vi "Omega DFG51-2 Force Gauge Logger.vi"() -> ()   [LabVIEW 2017]
uses:
  <vilib>/regexp/Match Regular Expression.xnode
  <vilib>/Analysis/NI_AALPro.lvlib
panel:
  out "after match":string
  out "before match":string
  in  "Tab Control":enum32{"Front Panel", "Save"}(tab)
  in  "Save?":bool=TRUE
  out "Realtime Plot":dbl(graph)
  out "Summary Plot":T1(graph)
  out "Device Response":string
  in  "Query to Device":string="?"
  in  "?":bool
  in  "Speed of Motor (cm/s)":dbl=0.01
  in  "COM Port":refnum<visa-resource-name>="COM5"
  out "Max Force":dbl format="%.4g"
  out "Integral of Force":dbl
  in  "Clear on Start":bool=TRUE
  out "Force vs. Displacement":cluster{"Get Start Time (s)":dbl, dbl, dbl[]}(graph)
  out "COM error out":errorcluster
  # "Molly's Palmer Stand = 0.01 cm/s = 6mm/min"
  # "Sample rate = 64 ms interval = 16Hz"
  # "8/31/2018\nMolly Roberts\n3/18/2015\nMatt George\nmngeorge@uw.edu"
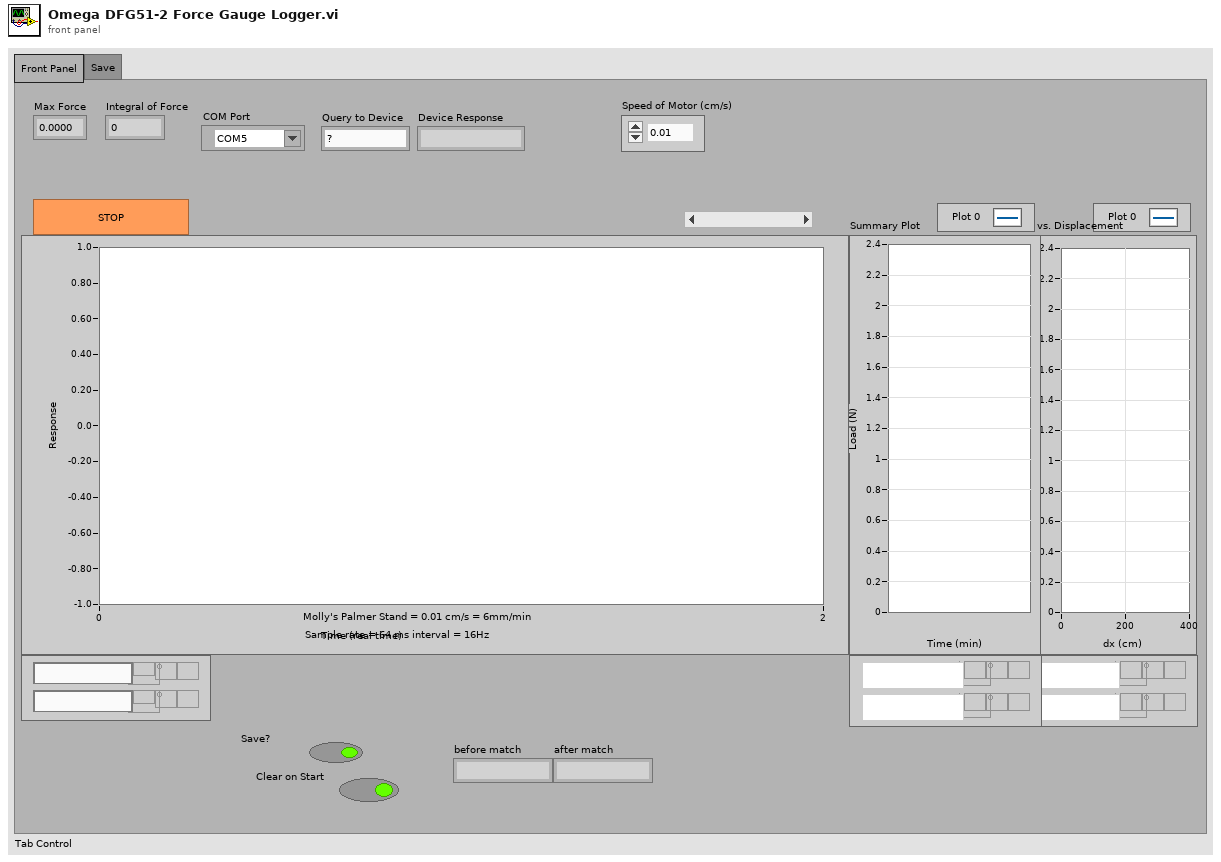
[diagram p1: front panel]
types:
  T1 = cluster{"Get Start Time (s)":dbl, "Sample rate (ms)":dbl, dbl[]}
  T2 = typedef "NI_Matrix.lvlib/RealMatrix.ctl" = dbl[][]
  T3 = enum16{"open", "replace", "create", "open or create", "replace or create", "replace or create with confirmation"}
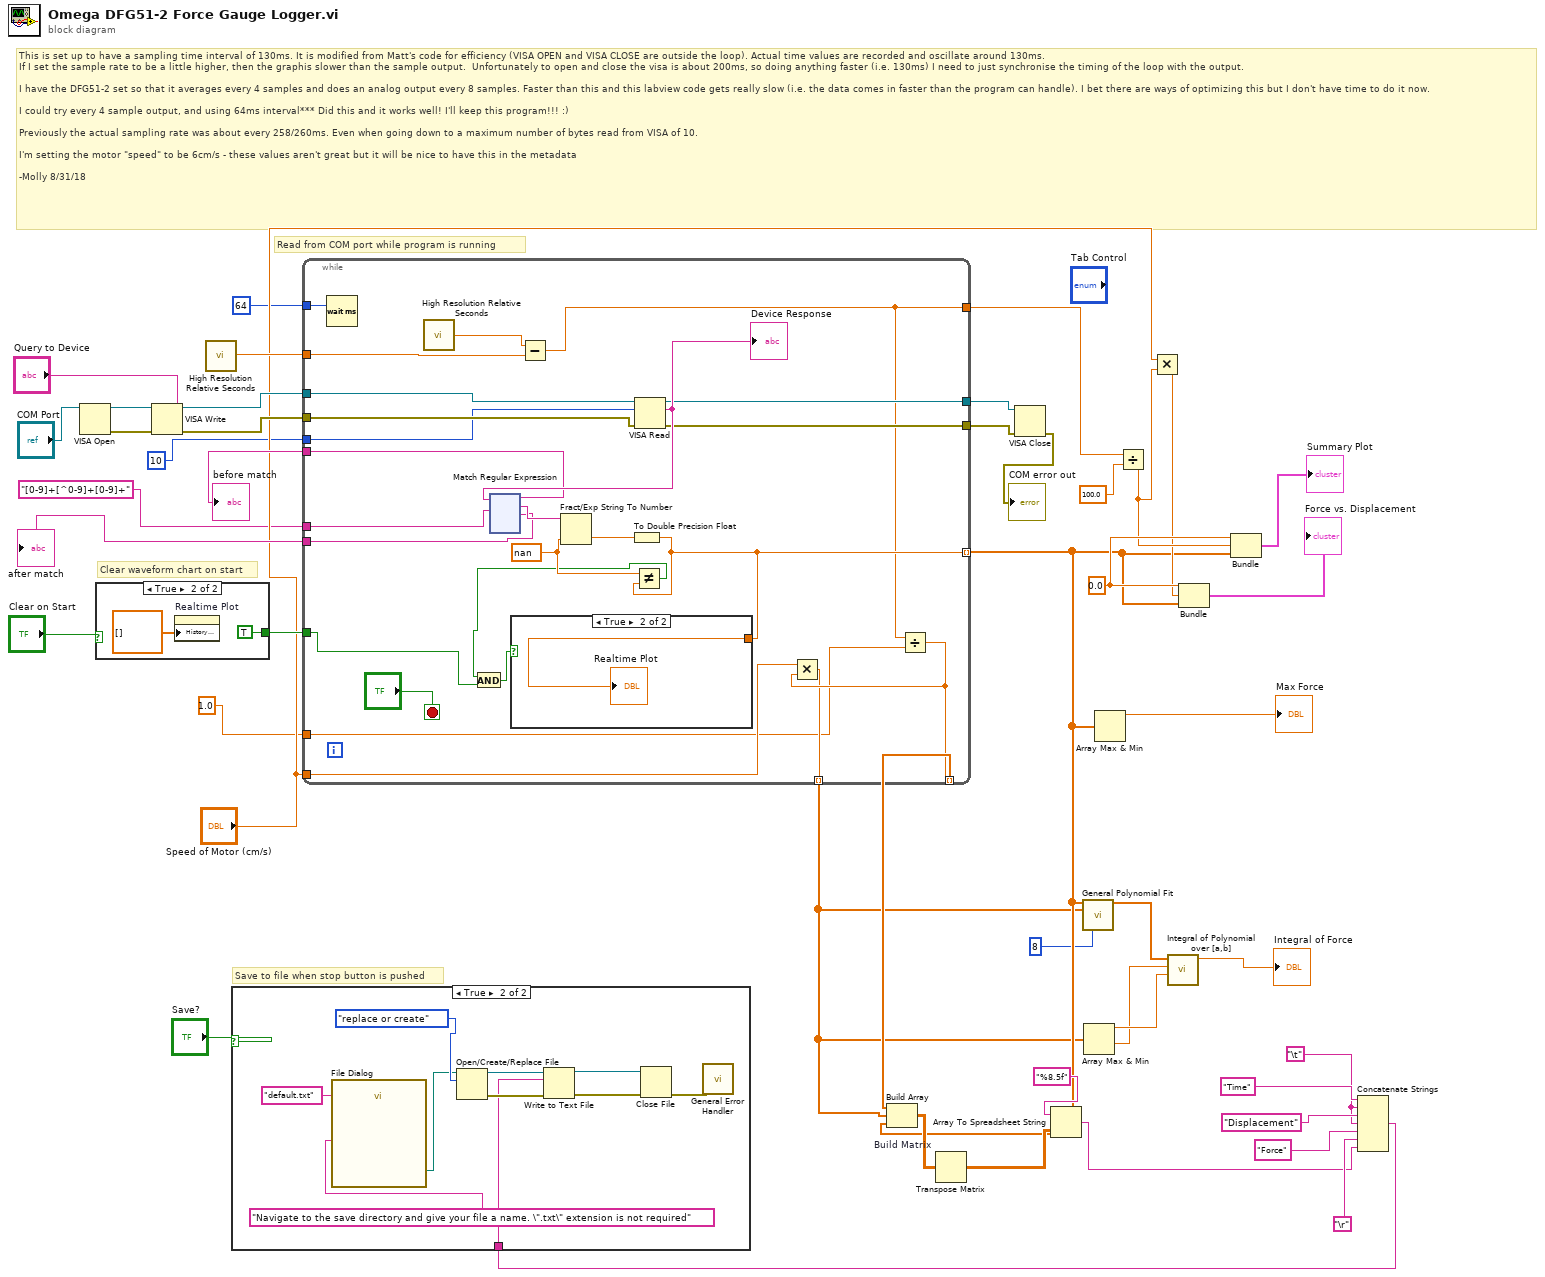
[diagram p0: block diagram]
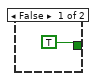
[diagram p2: hidden frame]
diagram:
  w35 = "\t"
  w45 = 0.0
  # "This is set up to have a sampling time interval of 130ms. It is modified from Matt's code for efficiency (VISA OPEN and VISA CLOSE are outside the loop). Actual time values are recorded and oscillate around 130ms. \nIf I set the sample rate to be a little higher, then the graphis slower than the sample output.  Unfortunately to open and close the visa is about 200ms, so doing anything faster (i.e. 130ms) I need to just synchronise the timing of the loop with the output. \n\nI have the DFG51-2 set so that it averages every 4 samples and does an analog output every 8 samples. Faster than this and this labview code gets really slow (i.e. the data comes in faster than the program can handle). I bet there are ways of optimizing this but I don't have time to do it now.\n\nI could try every 4 sample output, and using 64ms interval*** Did this and it works well! I'll keep this program!!! :)\n\nPreviously the actual sampling rate was about every 258/260ms. Even when going down to a maximum number of bytes read from VISA of 10. \n\nI'm setting the motor \"speed\" to be 6cm/s - these values aren't great but it will be nice to have this in the metadata\n\n-Molly 8/31/18"
  # "Clear waveform chart on start"
  # "Read from COM port while program is running"
  # "Save to file when stop button is pushed"
  n1 = VISA Open(VISA resource name="COM Port") -> (VISA resource name=w16:refnum<visa-resource-name>, error out=w18:errorcluster)  [unwired: 4 in]
  n2 = case shown="True" "Clear on Start" {
    tunnel: [TRUE TRUE] -> w8
    frame False {
    }
    frame True {
      n3 = property on="Realtime Plot" class="WFChart (strict)"("History Data"=dbl[] []) -> ()  [unwired: 2 in, 2 out]
    }
  }
  n4 = VISA Write(VISA resource name=w16, write buffer="Query to Device", error in (no error)=w18) -> (VISA resource name out=w14:refnum<visa-resource-name>, error out=w15:errorcluster)  [unwired: 1 out]
  n5 = call <vilib>:"High Resolution Relative Seconds.vi"() -> ("relative seconds"=w10:dbl)
  n6 = while {
    tunnel: [w67] -> w26 mode=indexing
    tunnel: [w60] -> w44
    tunnel: [w73] -> w32 mode=indexing
    tunnel: [w72] -> w23 mode=indexing
    tunnel: w15 -> [w66]
    tunnel: w14 -> [w65]
    tunnel: [w64] -> w13
    tunnel: [w63] -> w12
    tunnel: w10 -> [w61]
    tunnel: w8 -> [w57]
    tunnel: [w56] -> w7
    tunnel: [w55] -> w6
    tunnel: "Speed of Motor (cm/s)" -> [w54]
    tunnel: u32 10 ("byte count") -> [w53]
    tunnel: 1.0 ("y") -> [w52]
    tunnel: u32 64 ("milliseconds to wait") -> [w51]
    tunnel: "[0-9]+[^0-9]+[0-9]+" ("regular expression") -> [w50]
    stop <- "?" stop-if-true
    w68 = nan ("default (0 DBL)")
    n7 = Wait (ms)(milliseconds to wait=w51) -> ()  [unwired: 1 out]
    n8 = call <vilib>:"High Resolution Relative Seconds.vi"() -> ("relative seconds"=w62:dbl)
    n9 = Subtract(x=w62, y=w61) -> (x-y=w60:dbl)
    n10 = VISA Read(VISA resource name=w65, byte count=w53, error in (no error)=w66) -> (VISA resource name out=w63:refnum<visa-resource-name>, read buffer=w71:string, error out=w64:errorcluster)  [unwired: 1 out]
    "Device Response" <- w71
    n11 = xnode "Match Regular Expression"("input string"=w71, "regular expression"=w50) -> ("before match"=w56:string, "whole match"=w70:string, "after match"=w55:string)  [unwired: 4 in, 2 out]
    n12 = Fract/Exp String To Number(string=w70, default (0 dbl)=w68) -> (number=w69:dbl)  [unwired: 2 in, 1 out]
    n13 = To Double Precision Float(number=w69) -> (double precision float=w67:dbl)
    n14 = Not Equal?(x=w68, y=w67) -> (x != y?=w58:bool)
    n15 = And(x=w58, y=w57) -> (x .and. y?=w59:bool)
    n16 = case shown="True" w59 {
      tunnel: w67 -> [_ w75]
      frame False {
      }
      frame True {
        "Realtime Plot" <- w75
      }
    }
    n17 = Divide(x=w60, y=w52) -> (x/y=w73:dbl)
    n18 = Multiply(x=w54, y=w73) -> (x*y=w72:dbl)
  }
  "before match" <- w7
  "after match" <- w6
  n19 = Build Array "Build Matrix"(w32, w23, w26) -> (w31:T2)
  n20 = Transpose Matrix(1:w31) -> (0:w33:T2)
  n21 = VISA Close(VISA resource name=w12, error in (no error)=w13) -> (error out=→"COM error out":errorcluster)
  n22 = Array To Spreadsheet String(array=w33, 3:"%8.5f" ("format string")) -> (spreadsheet string=w30:string)  [unwired: 1 in]
  n23 = call <vilib>:"General Polynomial Fit.vi"("Y"=w26, "polynomial order"=8, "X"=w23) -> ("Best Polynomial Fit"=w24:dbl[])  [unwired: 9 in, 3 out]
  n24 = Array Max & Min(array=w23) -> (max value=w22:dbl, min value=w21:dbl)  [unwired: 2 out]
  n25 = Array Max & Min(array=w26) -> (max value=→"Max Force":dbl)  [unwired: 3 out]
  n26 = Divide(x=w44, y=100.0) -> (x/y=w42:dbl)
  n27 = Multiply(x="Speed of Motor (cm/s)", y=w42) -> (x*y=w41:dbl)
  n28 = call <vilib>:"Integral of Polynomial over [a,b].vi"("b"=w22, "a"=w21, "P(x)"=w24) -> ("integral of P(x)"=→"Integral of Force":dbl)  [unwired: 7 in, 1 out]
  n29 = Bundle(w45, w41, w26) -> (→"Force vs. Displacement":cluster{dbl, dbl, dbl[]})  [unwired: 1 in]
  n30 = Bundle(w45, w42, w26) -> (→"Summary Plot":cluster{dbl, dbl, dbl[]})  [unwired: 1 in]
  n31 = Concatenate Strings("Time" ("string"), w35, "Displacement" ("string"), w35, "Force" ("string"), "\r", w30) -> (w28:string)
  n32 = case shown="True" "Save?" {
    tunnel: w28 -> [_ w190]
    frame False {
    }
    frame True {
      n33 = call "File Dialog"("prompt"="Navigate to the save directory and give your file a name. \".txt\" extension is not required", "default name"="default.txt") -> ("selected path"=w189:path)  [unwired: 10 in, 3 out]
      n34 = Open/Create/Replace File(file path (use dialog)=w189, operation (0:open)=T3."replace or create") -> (refnum out=w191:refnum<file>, error out=w195:errorcluster)  [unwired: 4 in, 1 out]
      n35 = Write to Text File(file (use dialog)=w191, text=w190, error in=w195) -> (refnum out=w192:refnum<file>, error out=w194:errorcluster)  [unwired: 1 in, 1 out]
      n36 = Close File(refnum=w192, error in=w194) -> (error out=w193:errorcluster)  [unwired: 1 out]
      n37 = call <vilib>:"General Error Handler.vi"("error in (no error)"=w193) -> ()  [unwired: 10 in, 5 out]
    }
  }
